vi "[SubV]PID_Both.vi"(0 "Right Torque in":dbl, 1 "Kp_left":dbl, 2 "Kd_left":dbl, 4 "Assist":bool, 5 "Left Torque Desired":dbl, 6 "Right Torque Desired":dbl, 7 "Left Torque in":dbl, 9 "kp_right":dbl format="%#_13g", 11 "kd_right":dbl format="%#_13g") -> (14 "Right Torque":T2(graph), 15 "Left Torque":T1(graph), 18 "Right T Command":dbl, 19 "Left T Command":dbl)   [LabVIEW 2019]
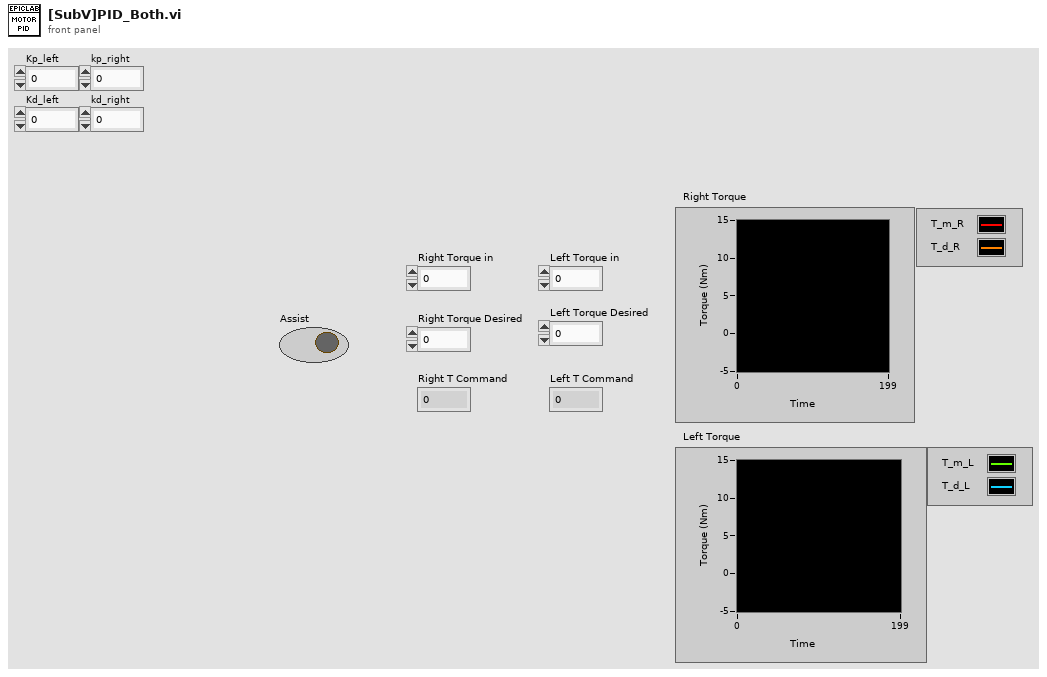
[diagram p1: front panel]
types:
  T1 = cluster{"Left Torque":dbl, "Left Desired Torque":dbl}
  T2 = cluster{"Right Torque in":dbl, "Right Torque Desired":dbl}
  T3 = cluster{"Left Torque in":dbl, "Left Torque Desired":dbl}
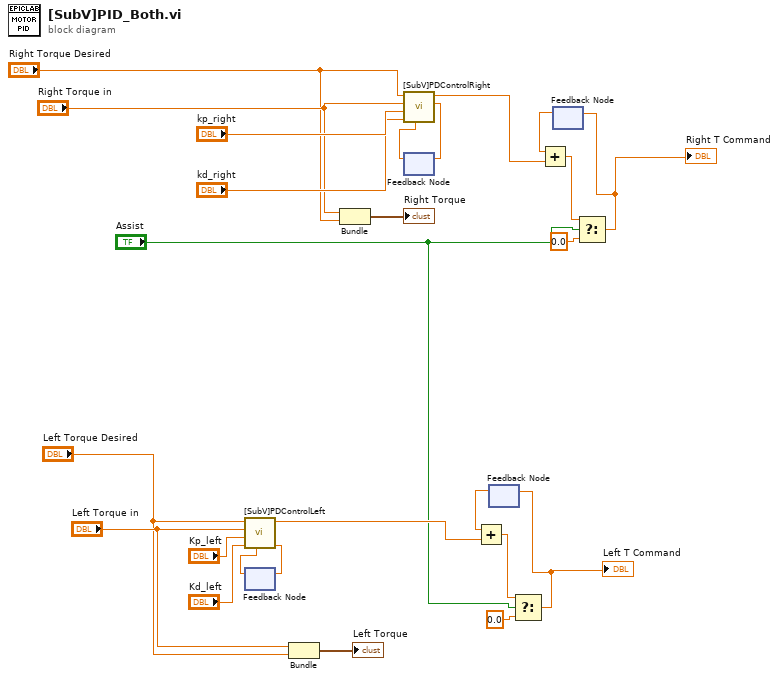
[diagram p0: block diagram]
diagram:
  n1 = feedback #1() -> (w22:dbl)  [unwired: 1 in]
  n2 = call "[SubV]PDControlLeft.vi"("Process Variable Old"=w22, "Kd"="Kd_left", "Kp"="Kp_left", "Process Variable"="Left Torque in", "Setpoint"="Left Torque Desired") -> ("Process Variable Out"=w21:dbl, "Left Out"=w3:dbl)  [unwired: 5 in]
  n3 = feedback-in #1(w21) -> ()
  n4 = Bundle("Left Torque in"="Left Torque in", "Left Torque Desired"="Left Torque Desired") -> (→"Left Torque":T3)  [unwired: 1 in]
  n5 = Bundle("Right Torque in"="Right Torque in", "Right Torque Desired"="Right Torque Desired") -> (→"Right Torque":T2)  [unwired: 1 in]
  n6 = feedback #2() -> (w24:dbl)  [unwired: 1 in]
  n7 = call "[SubV]PDControlRight.vi"("PV Old"=w24, "Kd"="kd_right", "Kp"="kp_right", "PV"="Right Torque in", "SP"="Right Torque Desired") -> ("PV Out"=w23:dbl, "Right Out"=w11:dbl)  [unwired: 5 in]
  n8 = feedback-in #2(w23) -> ()
  n9 = feedback #3() -> (w5:dbl)  [unwired: 1 in]
  n10 = Add(x=w5, y=w3) -> (x+y=w4:dbl)
  n11 = Select(t=w4, s="Assist", f=0.0) -> (s? t:f=w2:dbl)
  "Left T Command" <- w2
  n12 = feedback-in #3(w2) -> ()
  n13 = feedback #4() -> (w12:dbl)  [unwired: 1 in]
  n14 = Add(x=w12, y=w11) -> (x+y=w9:dbl)
  n15 = Select(t=w9, s="Assist", f=0.0) -> (s? t:f=w8:dbl)
  "Right T Command" <- w8
  n16 = feedback-in #4(w8) -> ()
